vi "Init Device.vi"(8 "error in (no error)":errorcluster, 11 "Laser Quantum in":refnum<class "Laser.lvclass">) -> (0 "error out":errorcluster, 3 "Laser Quantum out":refnum<class "Laser.lvclass">)   [LabVIEW 2018, in "Laser.lvlib" / "Laser.lvclass"]
uses:
  Laser.lvclass
  Laser.lvclass/Laser.ctl
  <vilib>/Instr/_visa.llb/VISA Configure Serial Port (Instr).vi
  Resources/GLOBAL/GLOBAL Debug.vi
  <vilib>/Utility/error.llb/Error Cluster From Error Code.vi
  <vilib>/ErrorRing/Error Ring.xnode
  Device/Device.lvclass
  Laser.lvlib
panel:
  out "VISA resource name out":refnum<visa-resource-name>
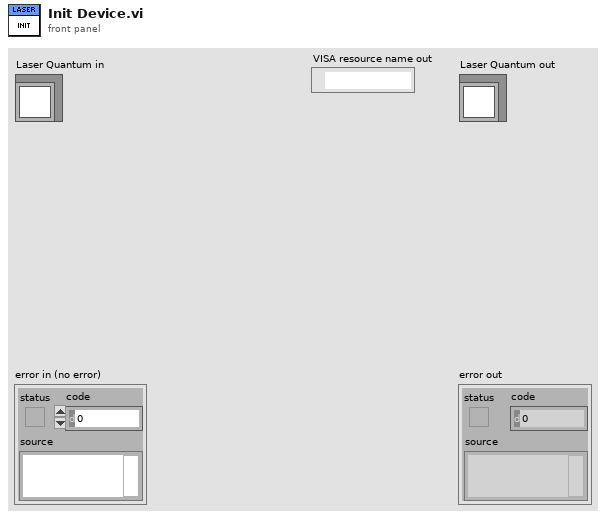
[diagram p1: front panel]
types:
  T1 = typedef "Laser Configuration.ctl" = cluster{"Serial Port":refnum<visa-resource-name>, "Laser Type":enum16{"Disable", "Laser Quantum", "Coherent OBIS", "PRM1-Z8", "Coherent HOPS"}, "Polarizer Amplitude":dbl, "Polarizer Theta Zero":dbl, "Wavelength":u16}
  T2 = enum16{"Disable", "Laser Quantum", "Coherent OBIS", "PRM1-Z8", "Coherent HOPS"}
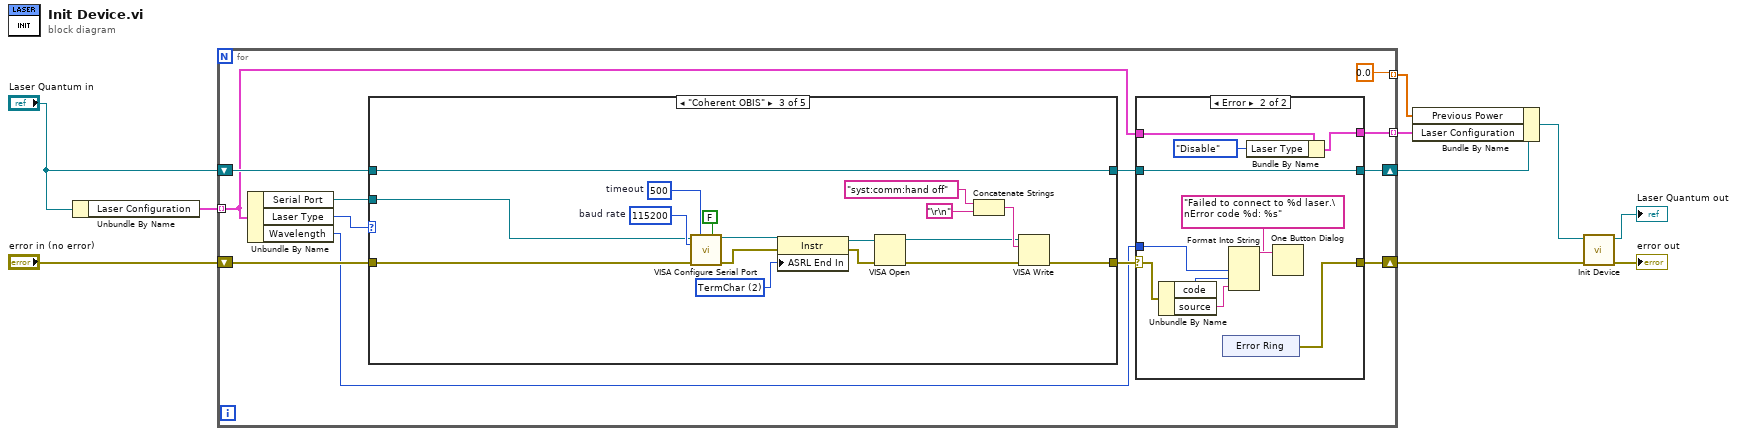
[diagram p0: block diagram]
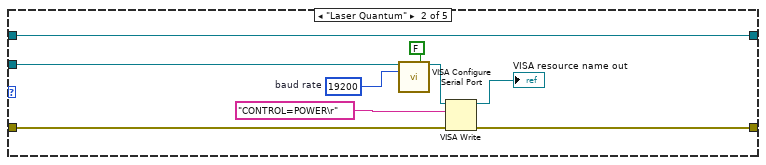
[diagram p4: hidden frame]
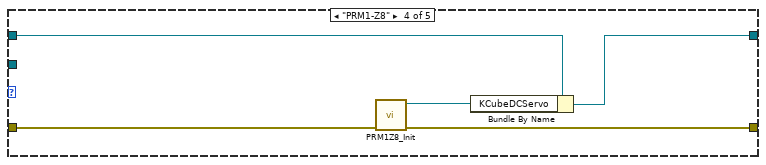
[diagram p5: hidden frame]
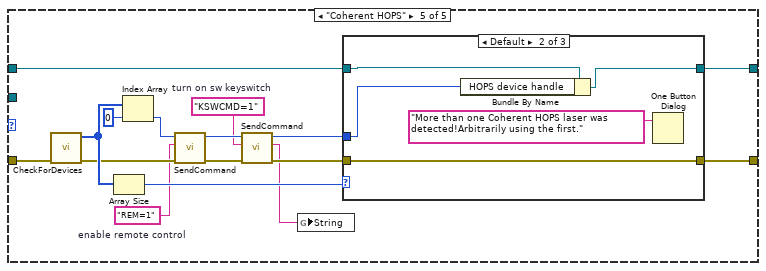
[diagram p6: hidden frame]
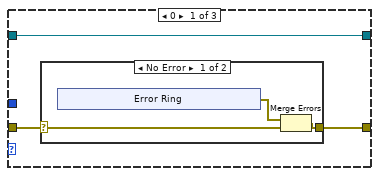
[diagram p7: hidden frame]
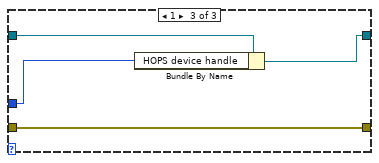
[diagram p9: hidden frame]
diagram:
  n1 = Unbundle By Name("Laser Quantum in") -> ("Laser Configuration"=w8:T1[])
  n2 = for {
    tunnel: w8 -> [w14] mode=indexing
    shift-right: [w17] -> w6
    shift-left: "error in (no error)" -> [w21]
    shift-right: [w15] -> w4
    shift-left: "Laser Quantum in" -> [w19]
    tunnel: [w13] -> w2 mode=indexing
    tunnel: [0.0] -> w1 mode=indexing
    n3 = Unbundle By Name(w14) -> ("Serial Port"=w22:refnum<visa-resource-name>, "Laser Type"=w20:T2, "Wavelength"=w12:u16)
    n4 = case shown="\"Coherent OBIS\"" w20 {
      tunnel: w22 -> [_ w47 w52 _ _]
      tunnel: w21 -> [w39 w43 w51 w70 w86]
      tunnel: [w39 w42 w60 w69 w82] -> w18
      tunnel: w19 -> [w38 w40 w59 w68 w81]
      tunnel: [w38 w40 w59 w67 w80] -> w16
      frame "Disable", Default {
      }
      frame "Laser Quantum" {
        w45 = u32 19200  # baud rate
        n5 = call-poly "VISA Configure Serial Port"("VISA resource name"=w47, "Enable Termination\nChar (T)"=FALSE ("Enable Termination\nChar (T)"), "baud rate (9600)"=w45) -> ("VISA resource name out"=w48:refnum<visa-resource-name>)  [unwired: 11 in, 1 out]
        n6 = VISA Write(VISA resource name=w48, write buffer="CONTROL=POWER\r", error in (no error)=w43) -> (VISA resource name out=→"VISA resource name out":refnum<visa-resource-name>, error out=w42:errorcluster)  [unwired: 1 out]
      }
      frame "Coherent OBIS" {
        w53 = u16 2 items=["None", "Last Bit", "TermChar"] ("Serial Settings:End Mode for Reads")
        w58 = u32 500  # timeout
        w61 = u32 115200  # baud rate
        n7 = call-poly "VISA Configure Serial Port"("VISA resource name"=w52, "timeout (10sec)"=w58, "Enable Termination\nChar (T)"=FALSE ("Enable Termination\nChar (T)"), "baud rate (9600)"=w61, "error in (no error)"=w51) -> ("VISA resource name out"=w57:refnum<visa-resource-name>, "error out"=w54:errorcluster)  [unwired: 9 in]
        n8 = property class="Instr"(reference=w57, error in=w54, "ASRL End In"=w53) -> (reference out=w56:refnum<visa-resource-name>, error out=w55:errorcluster)
        n9 = VISA Open(error in (no error)=w55, VISA resource name=w56) -> (VISA resource name=w49:refnum<visa-resource-name>, error out=w50:errorcluster)  [unwired: 3 in]
        n10 = Concatenate Strings("syst:comm:hand off" ("write to laser"), "\r\n") -> (w65:string)
        n11 = VISA Write(VISA resource name=w49, write buffer=w65, error in (no error)=w50) -> (error out=w60:errorcluster)  [unwired: 2 out]
      }
      frame "PRM1-Z8" {
        n12 = call "PRM1Z8_Init.vi"("error in (no error)"=w70) -> ("error out"=w69:errorcluster, "reference out"=w66:refnum<k24>)  [unwired: 9 in]
        n13 = Bundle By Name(cluster=w68, "KCubeDCServo"=w66) -> (w67:refnum<class "Laser.lvclass">)
      }
      frame "Coherent HOPS" {
        w71 = "KSWCMD=1"  # turn on sw keyswitch
        w77 = "REM=1"  # enable remote control
        n14 = call "CheckForDevices.vi"("error in"=w86) -> ("error out"=w79:errorcluster, "Device Handles"=w83:u64[])  [unwired: 6 in, 1 out]
        n15 = Array Size(array=w83) -> (size(s)=w84:i32)
        n16 = Index Array(array=w83, index=0 ("Index")) -> (element=w78:u64)
        n17 = call "SendCommand.vi"("error in"=w79, "Command"=w77, "Device Handle"=w78) -> ("error out"=w76:errorcluster, "Dup Handle"=w73:u64)  [unwired: 3 in, 2 out]
        n18 = call "SendCommand.vi"("error in"=w76, "Command"=w71, "Device Handle"=w73) -> ("error out"=w75:errorcluster, "String"=w72:string, "Dup Handle"=w74:u64)  [unwired: 3 in, 1 out]
        n19 = global write "GLOBAL Debug.vi" "String"(w72) -> ()
        n20 = case shown="Default" w84 {
          tunnel: w74 -> [_ w98 w103]
          tunnel: w75 -> [w87 w101 w106]
          tunnel: [w89 w101 w106] -> w82
          tunnel: w81 -> [w88 w99 w104]
          tunnel: [w88 w100 w105] -> w80
          frame 0 {
            n21 = case shown="No Error" w87 {
              selector: w87 -> [w90 w97]
              tunnel: [w92 w97] -> w89
              frame No Error {
                n22 = xnode "Error Ring"() -> ("error out"=w91:errorcluster)
                n23 = Merge Errors(w91, w90) -> (w92:errorcluster)
              }
              frame Error {
              }
            }
          }
          frame Default {
            n24 = Bundle By Name(cluster=w99, "HOPS device handle"=w98) -> (w100:refnum<class "Laser.lvclass">)
            n25 = One Button Dialog(message="More than one Coherent HOPS laser was detected!Arbitrarily using the first.") -> ()  [unwired: 1 in, 1 out]
          }
          frame 1 {
            n26 = Bundle By Name(cluster=w104, "HOPS device handle"=w103) -> (w105:refnum<class "Laser.lvclass">)
          }
        }
      }
    }
    n27 = case shown="Error" w18 {
      selector: w18 -> [w25 w31]
      tunnel: [w25 w36] -> w17
      tunnel: w16 -> [w24 w35]
      tunnel: [w24 w35] -> w15
      tunnel: w14 -> [w23 w34]
      tunnel: [w23 w33] -> w13
      tunnel: w12 -> [_ w26]
      frame No Error {
      }
      frame Error {
        n28 = Unbundle By Name(w31) -> ("code"=w27:i32, "source"=w28:string)
        n29 = xnode "Error Ring"() -> ("error out"=w36:errorcluster)
        n30 = Format Into String(format string="Failed to connect to %d laser.\nError code %d: %s" ("message"), w26, w27, w28) -> (resulting string=w30:string)  [unwired: 2 in, 1 out]
        n31 = Bundle By Name(cluster=w34, "Laser Type"=T2."Disable") -> (w33:T1)
        n32 = One Button Dialog(message=w30) -> ()  [unwired: 1 in, 1 out]
      }
    }
  }
  n33 = Bundle By Name(cluster=w4, "Previous Power"=w1, "Laser Configuration"=w2) -> (w3:refnum<class "Laser.lvclass">)
  n34 = call-parent "Init Device.vi"("error in (no error)"=w6, "Device in"=w3) -> ("error out"=→"error out":errorcluster, "Device out"=→"Laser Quantum out":refnum<class "Laser.lvclass">)  [unwired: 8 in]
